vi "Run Runnable.vi"(8 "error in (no error)":errorcluster, 10 "Runnable":refnum<class "Runnable.lvclass">, 11 "Test Runner":refnum<class "Parallell Test Runner.lvclass">) -> (0 "error out":errorcluster)   [LabVIEW 2020, in "Parallell Test Runner.lvclass"]
uses:
  Parallell Test Runner.lvclass
  Run/Runnable.lvclass
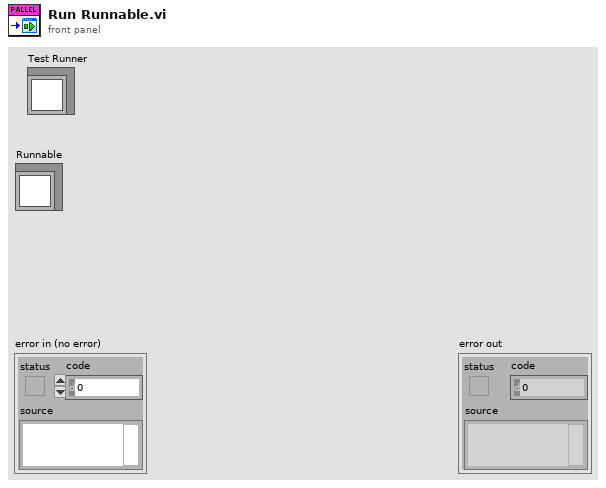
[diagram p1: front panel]
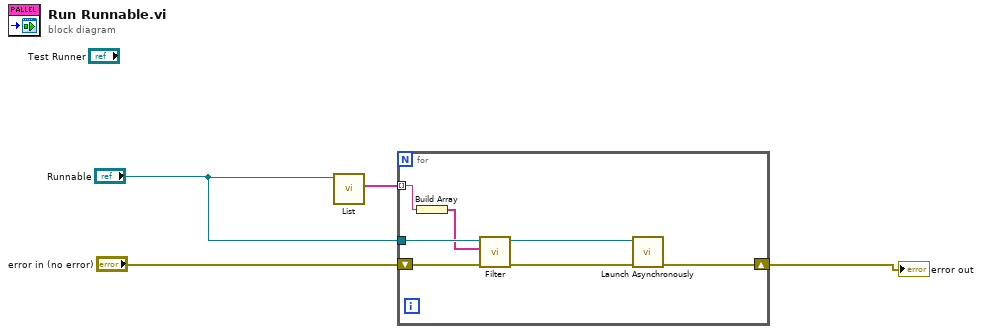
[diagram p0: block diagram]
diagram:
  n1 = call-dynamic "List.vi"("Runnable in"="Runnable") -> ("List of Runnables"=w4:string[])  [unwired: 9 in, 1 out]
  n2 = for {
    tunnel: w4 -> [w10] mode=indexing
    tunnel: "Runnable" -> [w11]
    shift-right: [w8] -> w1
    shift-left: "error in (no error)" -> [w7]
    n3 = Build Array(w10) -> (w9:string[])
    n4 = call-dynamic "Filter.vi"("error in (no error)"=w7, "Selected Runnables"=w9, "Runnable In"=w11) -> ("error out"=w6:errorcluster, "Runnable Out"=w5:refnum<class "Runnable.lvclass">)  [unwired: 7 in]
    n5 = call "Launch Asynchronously.vi"("error in (no error)"=w6, "Runnable in"=w5) -> ("error out"=w8:errorcluster)  [unwired: 9 in]
  }
  "error out" <- w1
